vi "Main.vi"(8 "error in":errorcluster, 11 "sequenceManagerWorker in":refnum<class "sequenceManagerWorker.lvclass">) -> (0 "error out":errorcluster, 3 "sequenceManagerWorker out":refnum<class "sequenceManagerWorker.lvclass">)   [LabVIEW 2023, in "sequenceManagerWorker.lvclass"]
doc: "The <b>Queued Message Handler</b> of the Worker that owns this VI."
uses:
  sequenceManagerWorker.lvclass
  Initialization Data.ctl
  Response Cases.ctl
  sequenceManagerWorker.lvclass/sequenceManagerWorker.ctl
  rqp_initializeManager.ctl
  ZE_Easy.Sequencer.lvlibp/SequenceManager/SequenceManager.lvclass
  rwr_getNexytStepsToExecute Reply.ctl
  ZE_Easy.Sequencer.lvlibp/Step/Step.lvclass
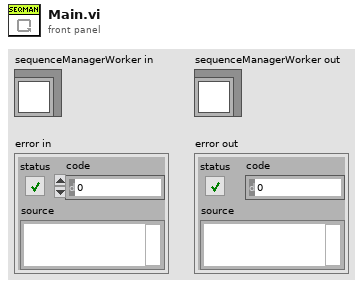
[diagram p1: front panel]
types:
  T1 = typedef "sequenceManagerWorker.lvclass/Initialization Data.ctl" = cluster{"Response Cases":T2}
  T2 = typedef "sequenceManagerWorker.lvclass/Response Cases.ctl" = cluster{"Placeholder - Can be deleted":string}
  T3 = typedef "sequenceManagerWorker.lvclass/rqp_initializeManager.ctl" = cluster{"Path to JSON sequence file":path}
  T4 = typedef "sequenceManagerWorker.lvclass/rwr_getNexytStepsToExecute Reply.ctl" = cluster{"StepsToExecuteInParallel":refnum<class "Step.lvclass">[]}
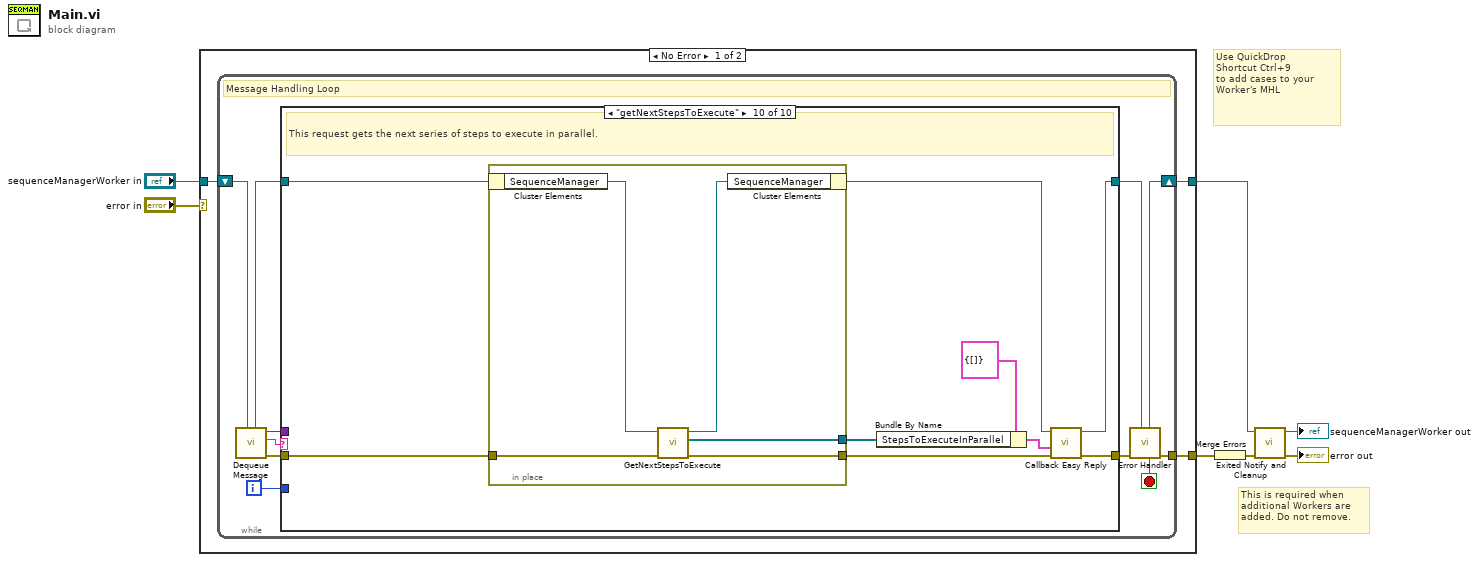
[diagram p0: block diagram]
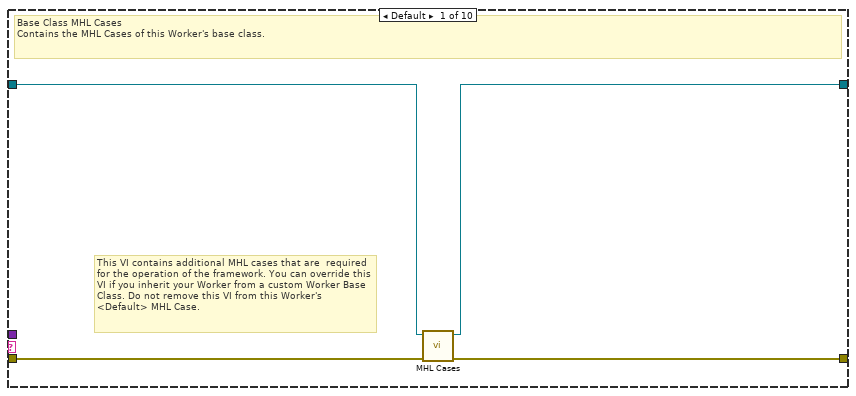
[diagram p2: hidden frame]
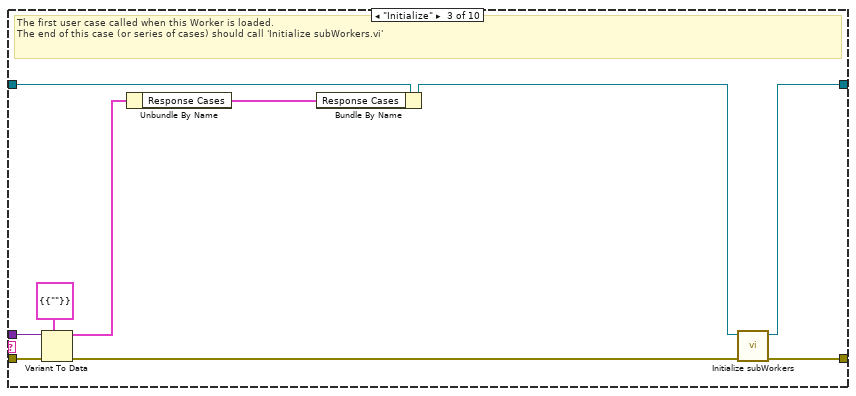
[diagram p4: hidden frame]
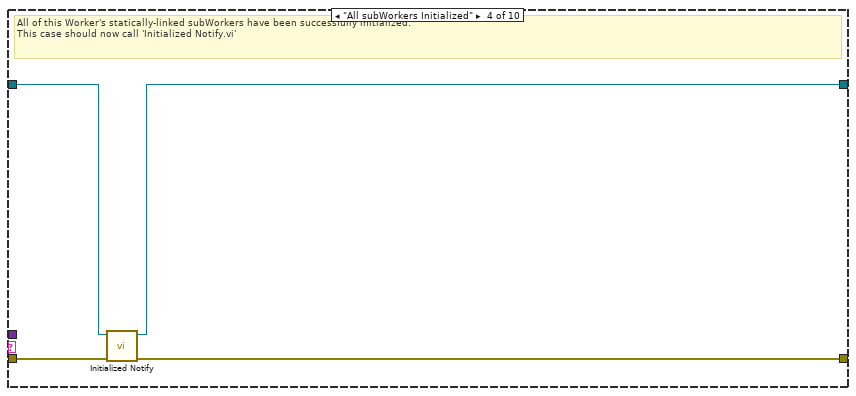
[diagram p5: hidden frame]
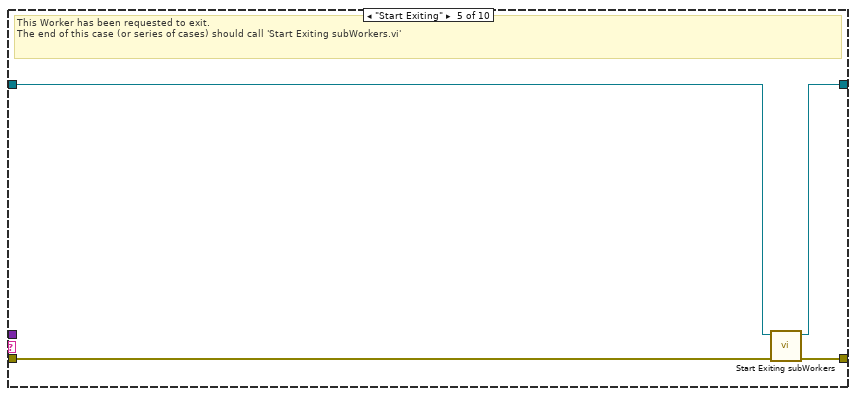
[diagram p6: hidden frame]
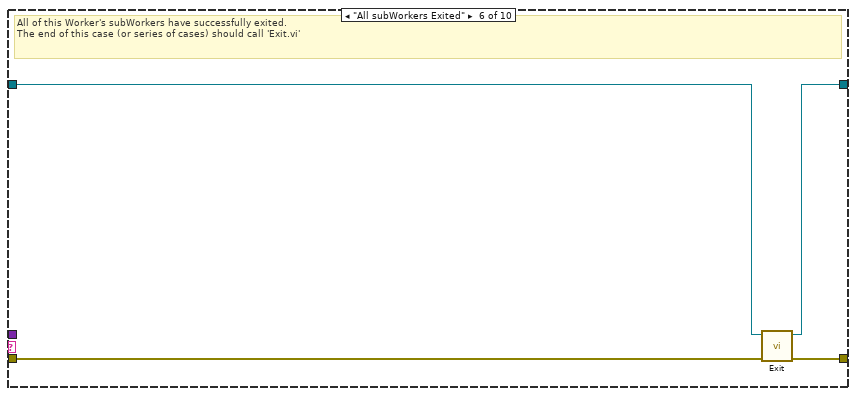
[diagram p7: hidden frame]
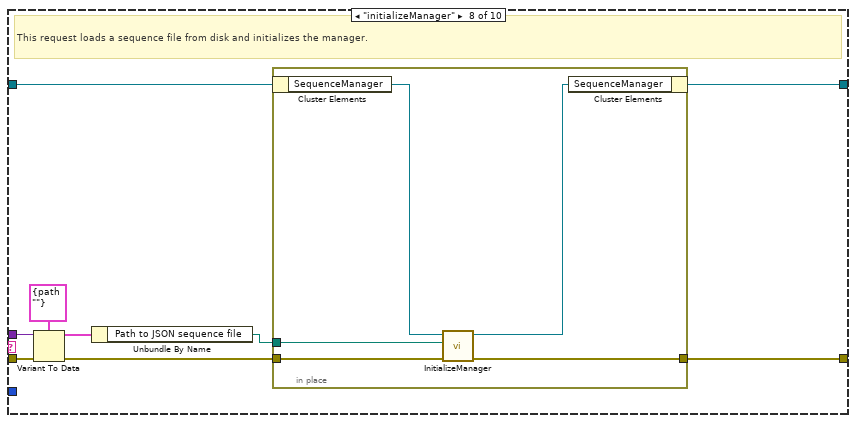
[diagram p9: hidden frame]
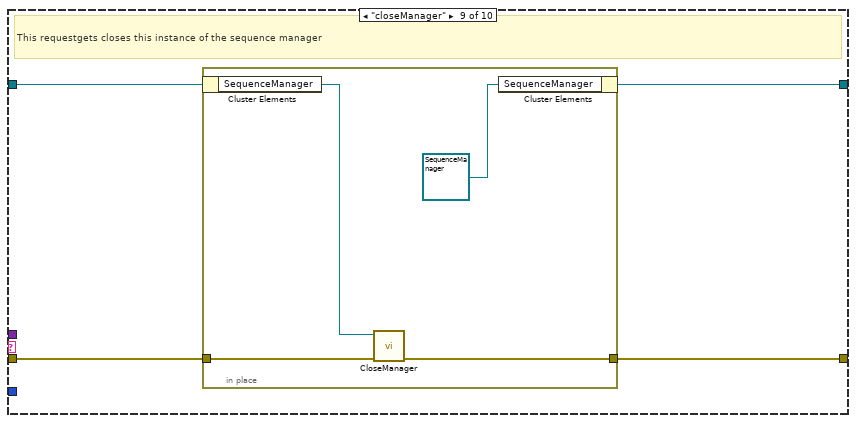
[diagram p10: hidden frame]
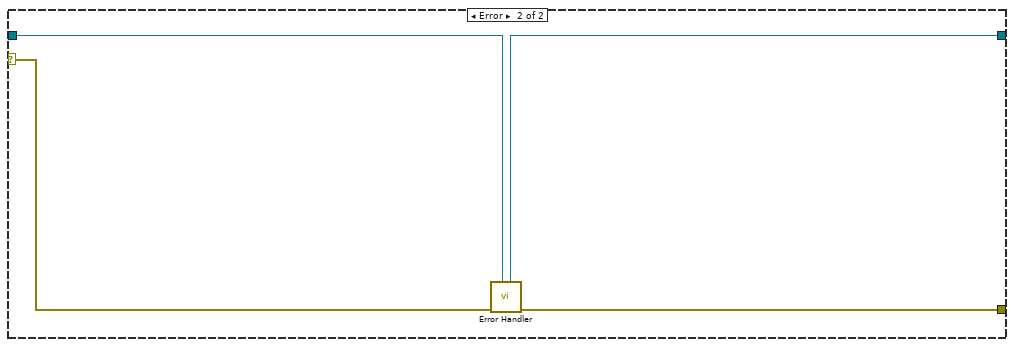
[diagram p11: hidden frame]
diagram:
  # "Use QuickDrop\nShortcut Ctrl+9\nto add cases to your\nWorker's MHL"
  # "This is required when additional Workers are added. Do not remove."
  n1 = case shown="No Error" "error in" {
    tunnel: "sequenceManagerWorker in" -> [w8 w89]
    tunnel: [w10 w90] -> w6
    tunnel: [w9 w88] -> w7
    selector: "error in" -> [_ w91]
    frame No Error {
      n2 = while {
        shift-right: [w19] -> w9
        shift-left: w8 -> [w21]
        tunnel: [w20] -> w10
        i -> [w12]
        stop <- w13 stop-if-true
        # "Message Handling Loop"
        n3 = call-dynamic "Dequeue Message.vi"("Worker"=w21) -> ("error out"=w18:errorcluster, "Case out"=w14:string, "Data out"=w11:variant, "Worker out"=w16:refnum<class "sequenceManagerWorker.lvclass">)  [unwired: 6 in, 1 out]
        n4 = case "Worker MHL Case Structure (DO NOT CHANGE LABEL NAME)" shown="\"getNextStepsToExecute\"" w14 {
          tunnel: w18 -> [w25 w26 w35 w41 w42 w49 w51 w60 w67 w77]
          tunnel: [w24 w26 w37 w40 w45 w48 w51 w54 w66 w82] -> w17
          tunnel: w16 -> [w23 w27 w34 w39 w43 w47 w50 w56 w69 w78]
          tunnel: [w22 w27 w36 w38 w44 w46 w50 w52 w68 w81] -> w15
          tunnel: w12 -> [_ _ _ _ _ _ _ _ _ _]
          tunnel: w11 -> [_ _ w32 _ _ _ _ w58 _ _]
          frame Default {
            # "This VI contains additional MHL cases that are  required for the operation of the framework. You can override this VI if you inherit your Worker from a custom Worker Base Class. Do not remove this VI from this Worker's <Default> MHL Case."
            # "Base Class MHL Cases\nContains the MHL Cases of this Worker's base class."
            n5 = call-dynamic "MHL Cases.vi"("error in"=w25, "Worker in"=w23) -> ("error out"=w24:errorcluster, "Worker out"=w22:refnum<class "sequenceManagerWorker.lvclass">)  [unwired: 8 in]
          }
          frame "------------ FRAMEWORK CASES -----------" {
            # "Start of Workers Framework Cases"
          }
          frame "Initialize" {
            # "The first user case called when this Worker is loaded.\nThe end of this case (or series of cases) should call 'Initialize subWorkers.vi'"
            n6 = Variant To Data(error in=w35, type=T1 {"Response Cases"={"Placeholder - Can be deleted"=""}} ("Cluster"), Variant=w32) -> (data=w30:T1, error out=w33:errorcluster)
            n7 = Unbundle By Name(w30) -> ("Response Cases"=w29:T2)
            n8 = Bundle By Name(cluster=w34, "Response Cases"=w29) -> (w31:refnum<class "sequenceManagerWorker.lvclass">)
            n9 = call-dynamic "Initialize subWorkers.vi"("error in"=w33, "Worker"=w31) -> ("error out"=w37:errorcluster, "dup Worker out"=w36:refnum<class "sequenceManagerWorker.lvclass">)  [unwired: 8 in]
          }
          frame "All subWorkers Initialized" {
            # "All of this Worker's statically-linked subWorkers have been successfully initialized.\nThis case should now call 'Initialized Notify.vi'"
            n10 = call-dynamic "Initialized Notify.vi"("error in"=w41, "Worker"=w39) -> ("error out"=w40:errorcluster, "dup Worker out"=w38:refnum<class "sequenceManagerWorker.lvclass">)  [unwired: 8 in]
          }
          frame "Start Exiting" {
            # "This Worker has been requested to exit. \nThe end of this case (or series of cases) should call 'Start Exiting subWorkers.vi'"
            n11 = call-dynamic "Start Exiting subWorkers.vi"("error_in"=w42, "Worker"=w43) -> ("error out"=w45:errorcluster, "dup Worker out"=w44:refnum<class "sequenceManagerWorker.lvclass">)  [unwired: 8 in]
          }
          frame "All subWorkers Exited" {
            # "All of this Worker's subWorkers have successfully exited. \nThe end of this case (or series of cases) should call 'Exit.vi'"
            n12 = call-dynamic "Exit.vi"("error_in"=w49, "Worker"=w47) -> ("error out"=w48:errorcluster, "dup Worker out"=w46:refnum<class "sequenceManagerWorker.lvclass">)  [unwired: 8 in]
          }
          frame "------------- PUBLIC API CASES -------------" {
            # "Start of Workers Public API Cases"
          }
          frame "initializeManager" {
            # "This request loads a sequence file from disk and initializes the manager."
            n13 = Variant To Data(error in=w60, type=T3 {"Path to JSON sequence file"=path ""} ("Data"), Variant=w58) -> (data=w57:T3, error out=w55:errorcluster)
            n14 = Unbundle By Name(w57) -> ("Path to JSON sequence file"=w53:path)
            n15 = in-place {
              in-place-border: w55 -> [w65]
              in-place-border: [w64] -> w54
              in-place-border: w53 -> [w61]
              n16 = in-place-cluster #1(w56) -> ("SequenceManager"=w63:refnum<class "SequenceManager.lvclass">)
              n17 = call-dynamic "InitializeManager.vi"("error in (no error)"=w65, "Path to JSON sequence file"=w61, "SequenceManager in"=w63) -> ("error out"=w64:errorcluster, "SequenceManager out"=w62:refnum<class "SequenceManager.lvclass">)  [unwired: 7 in]
              n18 = in-place-cluster #1("SequenceManager"=w62) -> (w52:refnum<class "sequenceManagerWorker.lvclass">)
            }
          }
          frame "closeManager" {
            # "This requestgets closes this instance of the sequence manager"
            n19 = in-place {
              in-place-border: w67 -> [w73]
              in-place-border: [w72] -> w66
              n20 = in-place-cluster #2(w69) -> ("SequenceManager"=w71:refnum<class "SequenceManager.lvclass">)
              n21 = call-dynamic "CloseManager.vi"("error in (no error)"=w73, "SequenceManager in"=w71) -> ("error out"=w72:errorcluster)  [unwired: 8 in, 1 out]
              n22 = in-place-cluster #2("SequenceManager"=refnum<class "SequenceManager.lvclass"> refnum) -> (w68:refnum<class "sequenceManagerWorker.lvclass">)
            }
          }
          frame "getNextStepsToExecute" {
            # "This request gets the next series of steps to execute in parallel."
            n23 = in-place {
              in-place-border: w77 -> [w85]
              in-place-border: [w84] -> w76
              in-place-border: [w83] -> w74
              n24 = in-place-cluster #3(w78) -> ("SequenceManager"=w87:refnum<class "SequenceManager.lvclass">)
              n25 = call-dynamic "GetNextStepsToExecute.vi"("error in (no error)"=w85, "SequenceManager in"=w87) -> ("error out"=w84:errorcluster, "Steps"=w83:refnum<class "Step.lvclass">[], "SequenceManager out"=w86:refnum<class "SequenceManager.lvclass">)  [unwired: 6 in, 1 out]
              n26 = in-place-cluster #3("SequenceManager"=w86) -> (w79:refnum<class "sequenceManagerWorker.lvclass">)
            }
            n27 = Bundle By Name(cluster=T4 {"StepsToExecuteInParallel"=[]} ("Reply Data"), "StepsToExecuteInParallel"=w74) -> (w75:T4)
            n28 = call-dynamic "Callback Easy Reply.vi"("error in"=w76, "Data"=w75, "Worker"=w79) -> ("error out"=w82:errorcluster, "dup Worker out"=w81:refnum<class "sequenceManagerWorker.lvclass">)  [unwired: 7 in]
          }
        }
        n29 = call-dynamic "Error Handler.vi"("Worker"=w15, "error_in"=w17) -> ("error out"=w20:errorcluster, "Stop Loop"=w13:bool, "Worker out"=w19:refnum<class "sequenceManagerWorker.lvclass">)  [unwired: 7 in]
      }
    }
    frame Error {
      n30 = call-dynamic "Error Handler.vi"("Worker"=w89, "error_in"=w91) -> ("error out"=w90:errorcluster, "Worker out"=w88:refnum<class "sequenceManagerWorker.lvclass">)  [unwired: 7 in, 1 out]
    }
  }
  n31 = Merge Errors(w6) -> (w3:errorcluster)
  n32 = call-dynamic "Exited Notify and Cleanup.vi"("error_in"=w3, "Worker"=w7) -> ("error out"=→"error out":errorcluster, "dup Worker out"=→"sequenceManagerWorker out":refnum<class "sequenceManagerWorker.lvclass">)  [unwired: 8 in]
